vi "HTTP-SetAuth.vi"(8 "error in (no error)":errorcluster, 11 "ByteGSWebAPI-V0 in":refnum<class "ByteGSWebAPI-V0.lvclass">) -> (0 "error out":errorcluster, 3 "ByteGSWebAPI-V0 out":refnum<class "ByteGSWebAPI-V0.lvclass">)   [LabVIEW 2019, in "ByteGSWebAPI-V0.lvclass"]
doc: "Setta l'header Authorization con il Token"
uses:
  ByteGSWebAPI-V0.lvclass
  ByteGSWebAPI-V0.lvclass/ByteGSWebAPI-V0.ctl
  <vilib>/httpClient/LabVIEWHTTPClient.lvlib
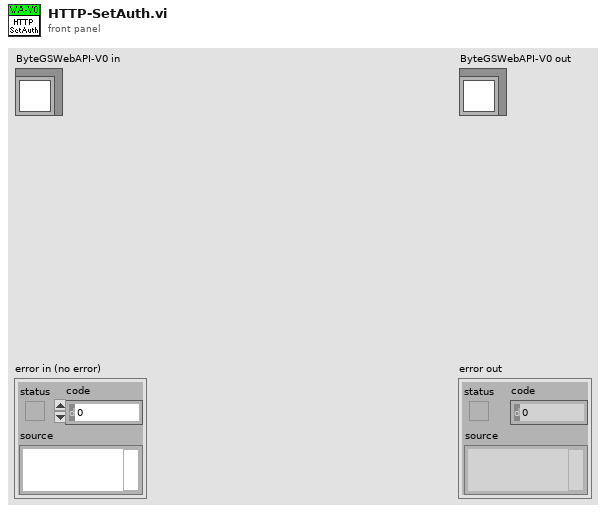
[diagram p1: front panel]
types:
  T1 = typedef "LabVIEWHTTPClient.lvlib/ClientHandle.ctl" = refnum<k1>
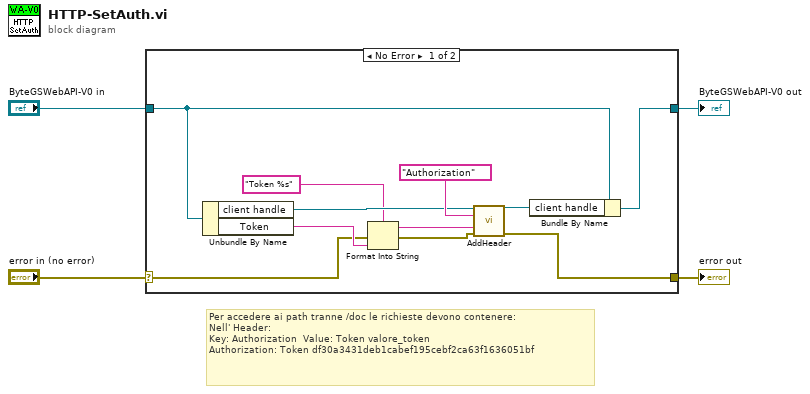
[diagram p0: block diagram]
diagram:
  # "Per accedere ai path tranne /doc le richieste devono contenere:\nNell' Header:\nKey: Authorization\t\tValue: Token valore_token\nAuthorization: Token df30a3431deb1cabef195cebf2ca63f1636051bf"
  n1 = case shown="No Error" "error in (no error)" {
    selector: "error in (no error)" -> [w6 w17]
    tunnel: [w12 w17] -> w3
    tunnel: [w11 w16] -> w1
    tunnel: "ByteGSWebAPI-V0 in" -> [w14 w16]
    frame No Error {
      n2 = Unbundle By Name(w14) -> ("client handle"=w13:T1, "Token"=w8:string)
      n3 = Format Into String(format string="Token %s", error in=w6, w8) -> (resulting string=w9:string, error out=w5:errorcluster)  [unwired: 1 in]
      n4 = call <vilib>:"AddHeader.vi"("client handle"=w13, "header"="Authorization", "value"=w9, "error in (no error)"=w5) -> ("client handle out"=w10:T1, "error out"=w12:errorcluster)  [unwired: 10 in]
      n5 = Bundle By Name(cluster=w14, "client handle"=w10) -> (w11:refnum<class "ByteGSWebAPI-V0.lvclass">)
    }
    frame Error {
    }
  }
  "error out" <- w3
  "ByteGSWebAPI-V0 out" <- w1
